vi "Click on tab.vi"(8 "error in (no error)":errorcluster) -> (0 "error out":errorcluster)   [LabVIEW 2011]
uses:
  user32.dll
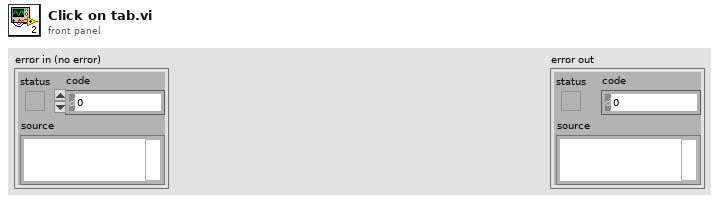
[diagram p1: front panel]
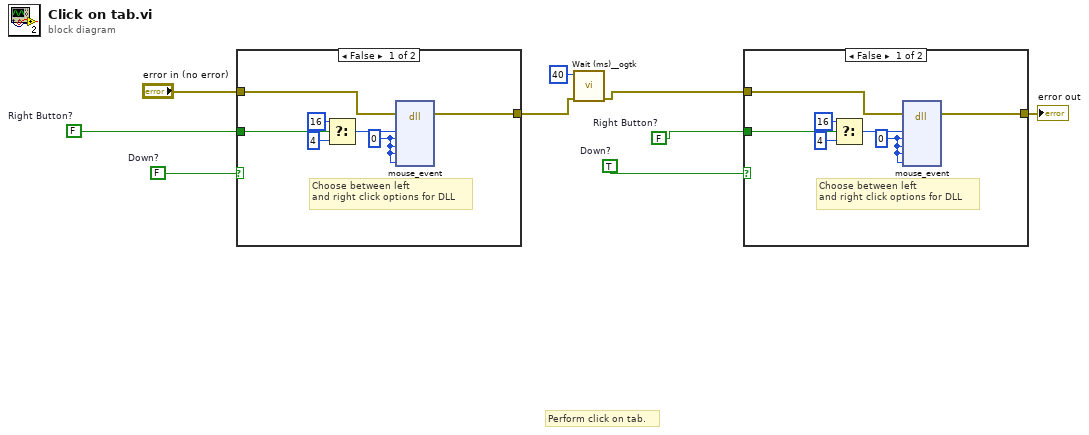
[diagram p0: block diagram]
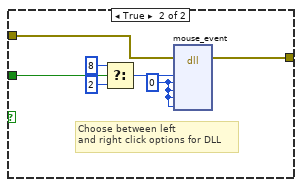
[diagram p2: hidden frame]
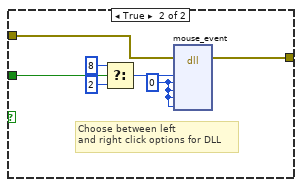
[diagram p3: hidden frame]
diagram:
  w7 = FALSE  # Down?
  w8 = FALSE  # Right Button?
  w3 = TRUE  # Down?
  w4 = FALSE  # Right Button?
  # "Perform click on tab."
  n1 = case shown="False" w7 {
    tunnel: w8 -> [w10 w23]
    tunnel: [w12 w22] -> w6
    tunnel: "error in (no error)" -> [w11 w21]
    frame False {
      w13 = 0 ("dx")
      # "Choose between left\nand right click options for DLL"
      n2 = Select(t=u32 16, s=w10, f=u32 4) -> (s? t:f=w16:u32)
      n3 = dll-call lib="user32.dll" fn="mouse_event"(error in=w11, "dwFlags"=w16, "dx"=w13, "dy"=w13, "dwData"=w13, "dwExtraInfo"=w13) -> (error out=w12:errorcluster)  [unwired: 7 in, 2 out]
    }
    frame True {
      w17 = 0 ("dx")
      # "Choose between left\nand right click options for DLL"
      n4 = Select(t=u32 8, s=w23, f=u32 2) -> (s? t:f=w20:u32)
      n5 = dll-call lib="user32.dll" fn="mouse_event"(error in=w21, "dwFlags"=w20, "dx"=w17, "dy"=w17, "dwData"=w17, "dwExtraInfo"=w17) -> (error out=w22:errorcluster)  [unwired: 7 in, 2 out]
    }
  }
  n6 = call <userlib>:"Wait (ms)__ogtk.vi"("error in (no error)"=w6, "milliseconds to wait"=u32 40) -> ("error out"=w5:errorcluster)  [unwired: 8 in, 1 out]
  n7 = case shown="False" w3 {
    tunnel: w4 -> [w24 w37]
    tunnel: [w26 w36] -> w1
    tunnel: w5 -> [w25 w35]
    frame False {
      w27 = 0 ("dx")
      # "Choose between left\nand right click options for DLL"
      n8 = Select(t=u32 16, s=w24, f=u32 4) -> (s? t:f=w30:u32)
      n9 = dll-call lib="user32.dll" fn="mouse_event"(error in=w25, "dwFlags"=w30, "dx"=w27, "dy"=w27, "dwData"=w27, "dwExtraInfo"=w27) -> (error out=w26:errorcluster)  [unwired: 7 in, 2 out]
    }
    frame True {
      w31 = 0 ("dx")
      # "Choose between left\nand right click options for DLL"
      n10 = Select(t=u32 8, s=w37, f=u32 2) -> (s? t:f=w34:u32)
      n11 = dll-call lib="user32.dll" fn="mouse_event"(error in=w35, "dwFlags"=w34, "dx"=w31, "dy"=w31, "dwData"=w31, "dwExtraInfo"=w31) -> (error out=w36:errorcluster)  [unwired: 7 in, 2 out]
    }
  }
  "error out" <- w1
